vi "MB MFC Valve Override.vi"(7 "Action":T2, 8 "error in (no error)":errorcluster, 9 "Override":T1, 11 "TCP Ref":refnum<k5>) -> (0 "error out":errorcluster, 1 "Override":T1, 3 "dup TCP Ref":refnum<k5>)   [LabVIEW 2011]
doc: "This VI reads or writes the valve override of an MKS Modbus MFC."
uses:
  Type Definitions/Modbus Action.ctl
  Type Definitions/Valve Override.ctl
  EtherNet.lib/Modbus/mb Ethernet.llb/MB Modbus Command.ctl
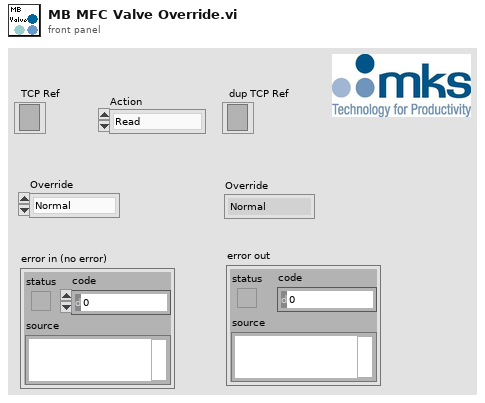
[diagram p1: front panel]
types:
  T1 = typedef "Valve Override.ctl" = enum16{"Normal", "Close", "Open"}
  T2 = typedef "Modbus Action.ctl" = enum16{"Read", "Write"}
  T3 = typedef "MB Modbus Command.ctl" = cluster{"Function Code":u8, "Starting Address":u16, "Quantity":u16, "Data":u16[], "Discrete":bool[]}
  T4 = typedef "MB Modbus Data Unit.ctl" = cluster{"Function Code":u8, "Data":u8[]}
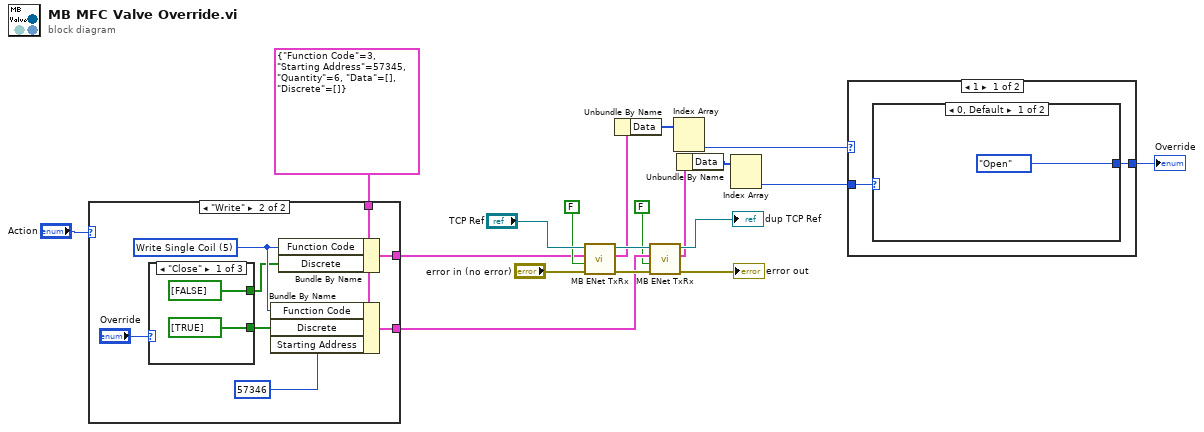
[diagram p0: block diagram]
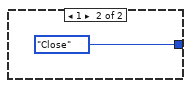
[diagram p2: hidden frame]
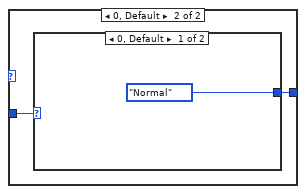
[diagram p3: hidden frame]
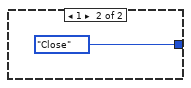
[diagram p4: hidden frame]
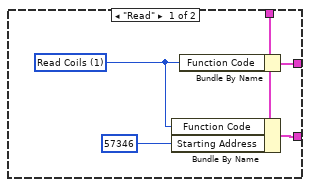
[diagram p5: hidden frame]
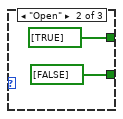
[diagram p6: hidden frame]
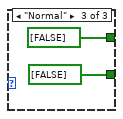
[diagram p7: hidden frame]
diagram:
  n1 = case shown="\"Write\"" "Action" {
    tunnel: T3 {"Function Code"=3, "Starting Address"=57345, "Quantity"=6, "Data"=[], "Discrete"=[]} ("Modbus Command") -> [w21 w29]
    tunnel: [w24 w32] -> w10
    tunnel: [w23 w30] -> w9
    frame "Read" {
      w22 = u8 1 items=["Read Coils"=1, "Read Discrete Inputs"=2, "Read Holding Registers"=3, "Read Input Registers"=4, "Write Single Coil"=5, "Write Single Register"=6, "Read Exception Status"=7, "Write Multiple Coils"=15, "Write Multiple Registers"=16, "Read Device Id"=43] ("Function Code")
      n2 = Bundle By Name(cluster=w21, "Function Code"=w22, "Starting Address"=u16 57346) -> (w23:T3)
      n3 = Bundle By Name(cluster=w21, "Function Code"=w22) -> (w24:T3)
    }
    frame "Write" {
      w28 = u8 5 items=["Read Coils"=1, "Read Discrete Inputs"=2, "Read Holding Registers"=3, "Read Input Registers"=4, "Write Single Coil"=5, "Write Single Register"=6, "Read Exception Status"=7, "Write Multiple Coils"=15, "Write Multiple Registers"=16, "Read Device Id"=43] ("Function Code")
      n4 = case shown="\"Close\"" "Override" {
        tunnel: [bool[] [FALSE] ("Discrete") bool[] [TRUE] ("Discrete") bool[] [FALSE] ("Discrete")] -> w26
        tunnel: [bool[] [TRUE] ("Discrete") bool[] [FALSE] ("Discrete") bool[] [FALSE] ("Discrete")] -> w25
        frame "Close" {
        }
        frame "Open" {
        }
        frame "Normal" {
        }
      }
      n5 = Bundle By Name(cluster=w29, "Function Code"=w28, "Discrete"=w25, "Starting Address"=u16 57346) -> (w30:T3)
      n6 = Bundle By Name(cluster=w29, "Function Code"=w28, "Discrete"=w26) -> (w32:T3)
    }
  }
  n7 = call "MB ENet TxRx.vi"("error in (no error)"="error in (no error)", "Use MODBUS Data Unit?"=FALSE, "Modbus Command"=w10, "TCP Ref:ValBlock"="TCP Ref") -> ("error out"=w15:errorcluster, "Modbus Data Unit Out"=w7:T4, "dup TCP Ref:ValBlock"=w12:refnum<k5>)  [unwired: 3 in, 2 out]
  n8 = Unbundle By Name(w7) -> ("Data"=w5:u8[])
  n9 = call "MB ENet TxRx.vi"("error in (no error)"=w15, "Use MODBUS Data Unit?"=FALSE, "Modbus Command"=w9, "TCP Ref:ValBlock"=w12) -> ("error out"=→"error out":errorcluster, "Modbus Data Unit Out"=w6:T4, "dup TCP Ref:ValBlock"=→"dup TCP Ref":refnum<k5>)  [unwired: 3 in, 2 out]
  n10 = Index Array(array=w5) -> (element #2=w4:u8)  [unwired: 2 in, 1 out]
  n11 = Unbundle By Name(w6) -> ("Data"=w3:u8[])
  n12 = Index Array(array=w3) -> (element #2=w2:u8)  [unwired: 2 in, 1 out]
  n13 = case shown="1" w4 {
    tunnel: w2 -> [w40 w44]
    tunnel: [w39 w43] -> w8
    frame 1 {
      n14 = case shown="0, Default" w40 {
        tunnel: [Valve_Override."Open" ("Override") Valve_Override."Close" ("Override")] -> w39
        frame 0, Default {
        }
        frame 1 {
        }
      }
    }
    frame 0, Default {
      n15 = case shown="0, Default" w44 {
        tunnel: [Valve_Override."Normal" ("Override") Valve_Override."Close" ("Override")] -> w43
        frame 0, Default {
        }
        frame 1 {
        }
      }
    }
  }
  "Override" <- w8
